vi "adjust_AI_range.vi"(8 "error in (no error)":errorcluster, 11 "DAQ task (in)":refnum<k21>) -> (0 "error out":errorcluster, 3 "DAQ task (out)":refnum<k21>, 4 "U.Max":dbl, 5 "Ush.Max":dbl, 6 "U.Min":dbl, 7 "Ush.Min":dbl)   [LabVIEW 2017]
uses:
  <vilib>/DAQmx/read.llb/DAQmx Read (Analog 2D DBL NChan NSamp).vi
  <vilib>/DAQmx/miscellaneous.llb/DAQmx Fill In Error Info.vi
  <resource>/objmgr/daqmx.rc
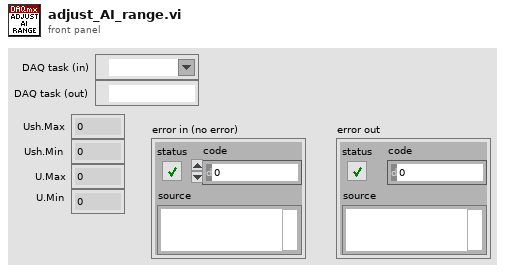
[diagram p1: front panel]
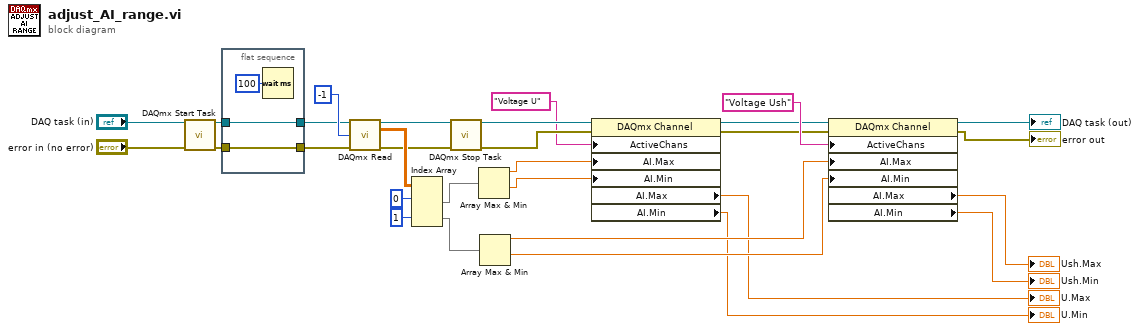
[diagram p0: block diagram]
diagram:
  n1 = call <vilib>:"DAQmx Start Task.vi"("task/channels in"="DAQ task (in)", "error in"="error in (no error)") -> ("task out"=w12:refnum<k21>, "error out"=w14:errorcluster)  [unwired: 12 in]
  n2 = flat-sequence {
    tunnel: w14 -> [w33]
    tunnel: [w33] -> w13
    tunnel: w12 -> [w32]
    tunnel: [w32] -> w11
    frame #0 {
      n3 = Wait (ms)(milliseconds to wait=u32 100) -> ()  [unwired: 1 out]
    }
  }
  n4 = call-poly <vilib>:"DAQmx Read.vi"("task/channels in"=w11, "number of samples per channel"=-1, "error in"=w13) -> ("task out"=w17:refnum<k21>, "data"=w18:dbl[][], "error out"=w16:errorcluster)  [unwired: 10 in]
  n5 = Index Array(array=w18, index (row) #1=0 ("index"), index (row) #2=1 ("index")) -> (element #1=w10:dbl[], element #2=w9:dbl[])  [unwired: 2 in]
  n6 = call <vilib>:"DAQmx Stop Task.vi"("task/channels in"=w17, "error in"=w16) -> ("task out"=w21:refnum<k21>, "error out"=w22:errorcluster)  [unwired: 12 in]
  n7 = Array Max & Min(array=w10) -> (max value=w23:dbl, min value=w24:dbl)  [unwired: 2 out]
  n8 = Array Max & Min(array=w9) -> (max value=w25:dbl, min value=w26:dbl)  [unwired: 2 out]
  n9 = property class="DAQmx Channel"(reference=w21, error in=w22, "ActiveChans"="Voltage U", "AI.Max"=w23, "AI.Min"=w24) -> (reference out=w1:refnum<k21>, error out=w2:errorcluster, "AI.Max"=→"U.Max":dbl, "AI.Min"=→"U.Min":dbl)
  n10 = property class="DAQmx Channel"(reference=w1, error in=w2, "ActiveChans"="Voltage Ush", "AI.Max"=w25, "AI.Min"=w26) -> (reference out=→"DAQ task (out)":refnum<k21>, error out=→"error out":errorcluster, "AI.Max"=→"Ush.Max":dbl, "AI.Min"=→"Ush.Min":dbl)
